vi "Write Connection Lookup.vi"(8 "error in (no error)":errorcluster, 10 "Routing Templates.lvlib:Abstract Connection Lookup.lvclass":refnum<class "Abstract Connection Lookup.lvclass">, 11 "Abstract Routing Channel Template in":refnum<class "Abstract Routing Channel Template.lvclass">) -> (0 "error out":errorcluster, 3 "Abstract Routing Channel Template out":refnum<class "Abstract Routing Channel Template.lvclass">)   [LabVIEW 2020, in "Routing Templates.lvlib" / "Abstract Routing Channel Template.lvclass"]
uses:
  Abstract Routing Channel Template.lvclass
  Abstract Routing Channel Template.lvclass/Abstract Routing Channel Template.ctl
  Connection Lookups/Abstract Connection Lookup/Abstract Connection Lookup.lvclass
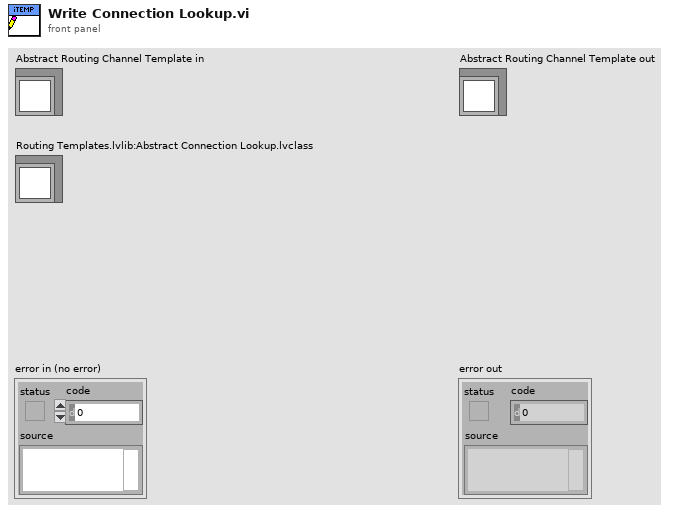
[diagram p1: front panel]
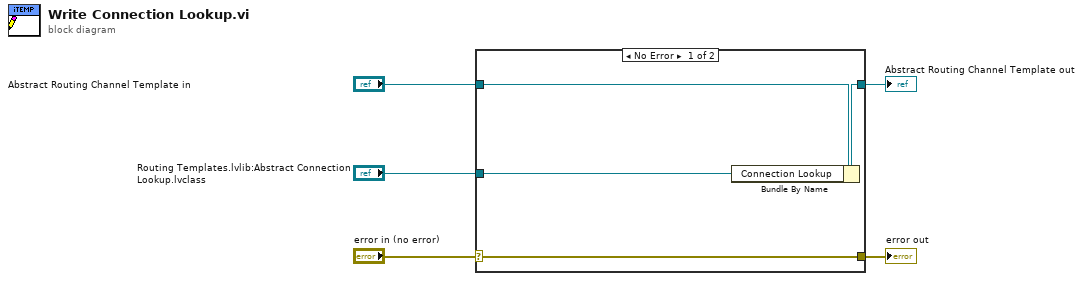
[diagram p0: block diagram]
diagram:
  n1 = case shown="No Error" "error in (no error)" {
    selector: "error in (no error)" -> [w9 w10]
    tunnel: [w9 w10] -> w4
    tunnel: [w7 w11] -> w2
    tunnel: "Abstract Routing Channel Template in" -> [w8 w11]
    tunnel: "Routing Templates.lvlib:Abstract Connection Lookup.lvclass" -> [w6 _]
    frame No Error {
      n2 = Bundle By Name(cluster=w8, "Connection Lookup"=w6) -> (w7:refnum<class "Abstract Routing Channel Template.lvclass">)
    }
    frame Error {
    }
  }
  "error out" <- w4
  "Abstract Routing Channel Template out" <- w2
